vi "4461 Replace AO Ch.vi"(8 "error in (no error)":errorcluster, 10 "Lockin (NEW)":refnum<class "Instrument.Lockin.lvclass">, 11 "Lockin (OLD)":refnum<class "Instrument.Lockin.lvclass">) -> (0 "error out":errorcluster, 1 "Ref different?":bool, 2 "AO different?":bool, 3 "Lockin out":refnum<class "Instrument.Lockin.lvclass">)   [LabVIEW 2016, in "Instrument.Lockin.lvclass"]
uses:
  Instrument.Lockin.lvclass
  Instrument.Lockin.lvclass/Instrument.Lockin.ctl
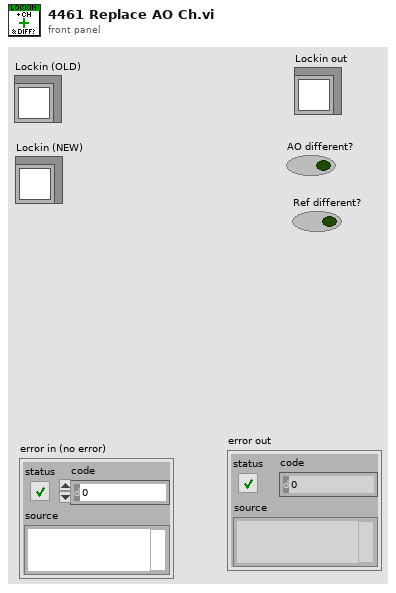
[diagram p1: front panel]
types:
  T1 = typedef "Instrument.Lockin.lvclass/AO-cluster.ctl" = cluster{"AO Amp (V)":T2, "AO DC (V)":T3, "AO f (Hz)":T4, "AO Phase (°)":T5, "Function":T6, "I+":bool[], "Sweeping":bool[]}
  T2 = typedef "Instrument.Lockin.lvclass/AO_Amp-array.ctl" = dbl[]
  T3 = typedef "Instrument.Lockin.lvclass/AO_DC-array.ctl" = dbl[]
  T4 = typedef "Instrument.Lockin.lvclass/AO_f-array.ctl" = dbl[]
  T5 = typedef "Instrument.Lockin.lvclass/AO_phi-array.ctl" = dbl[]
  T6 = typedef "Instrument.Lockin.lvclass/Function-array.ctl" = T7[]
  T7 = typedef "Instrument.Lockin.lvclass/Function-enum.ctl" = enum16{"Sine", "Triangle", "Square", "Sawtooth"}
  T8 = typedef "Instrument.Lockin.lvclass/REF-cluster.ctl" = cluster{"REF f (Hz)":T9, "REF phi (°)":T10}
  T9 = typedef "Instrument.Lockin.lvclass/REF_f-array.ctl" = dbl[]
  T10 = typedef "Instrument.Lockin.lvclass/REF_phi-array.ctl" = dbl[]
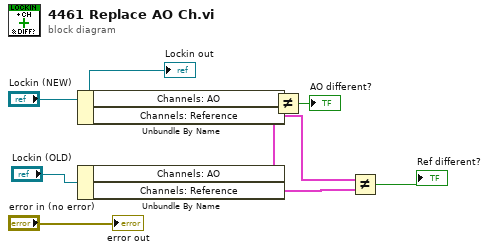
[diagram p0: block diagram]
diagram:
  n1 = Unbundle By Name("Lockin (NEW)") -> ("Channels: AO"=w6:T1, "Channels: Reference"=w3:T8)
  n2 = Unbundle By Name("Lockin (OLD)") -> ("Channels: AO"=w8:T1, "Channels: Reference"=w2:T8)
  n3 = Not Equal?(x=w6, y=w8) -> (x != y?=→"AO different?":bool)
  n4 = Not Equal?(x=w3, y=w2) -> (x != y?=→"Ref different?":bool)
  "Lockin out" <- "Lockin (NEW)"
  "error out" <- "error in (no error)"
